vi "Save Settings.vi"(7 "XML File Path":path, 8 "error in (no error)":errorcluster, 10 "Reader Object":refnum<class>, 11 "Scanner Object":refnum<class>) -> (0 "error out":errorcluster)   [LabVIEW 2017, in "File IO.lvclass"]
uses:
  File IO/File IO.lvclass
  Scanners/Scanner/Write Range UI.vi
  File IO/Setup UI.vi
  <vilib>/Utility/xml.llb/Write to XML File(string).vi
  Scanners/Scanner/Scanner.lvclass
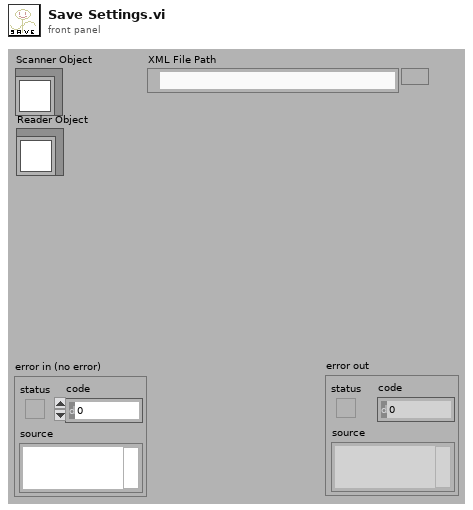
[diagram p1: front panel]
types:
  T1 = cluster{"output cluster":cluster{i32[][], string[]}, "output cluster":cluster{i32[][], string[]}, "output cluster":cluster{i32[][], string[]}, "output cluster":cluster{i32[][], string[]}}
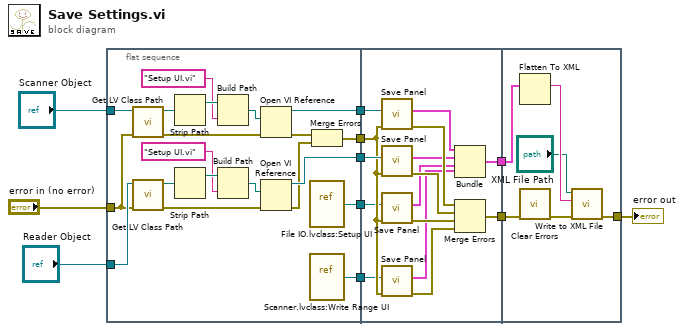
[diagram p0: block diagram]
diagram:
  n1 = flat-sequence {
    tunnel: "Scanner Object" -> [w29]
    tunnel: "Reader Object" -> [w31]
    tunnel: "error in (no error)" -> [w30]
    tunnel: [w28] -> w10
    tunnel: [w27] -> w9
    tunnel: [w26] -> w8
    tunnel: [w23] -> w7
    tunnel: [w22] -> w3
    tunnel: w10 -> [w46]
    tunnel: w9 -> [w45]
    tunnel: w8 -> [w44]
    tunnel: w7 -> [w43]
    tunnel: [w38] -> w6
    tunnel: [w33] -> w5
    tunnel: w3 -> [w32]
    tunnel: w6 -> [w52]
    tunnel: w5 -> [w51]
    tunnel: [w50] -> w4
    frame #0 {
      n2 = call <vilib>:"Get LV Class Path.vi"("error in (no error)"=w30, "object"=w29) -> ("error out"=w17:errorcluster, "class path"=w21:path)  [unwired: 8 out]
      n3 = call <vilib>:"Get LV Class Path.vi"("error in (no error)"=w30, "object"=w31) -> ("error out"=w12:errorcluster, "class path"=w16:path)  [unwired: 8 out]
      n4 = Strip Path(path=w21) -> (stripped path=w20:path)  [unwired: 1 out]
      n5 = Strip Path(path=w16) -> (stripped path=w15:path)  [unwired: 1 out]
      n6 = Build Path(base path=w20, name or relative path="Setup UI.vi") -> (appended path=w18:path)
      n7 = Build Path(base path=w15, name or relative path="Setup UI.vi") -> (appended path=w13:path)
      n8 = Open VI Reference(vi path=w18, error in (no error)=w17) -> (vi reference=w28:refnum<vi>, error out=w25:errorcluster)  [unwired: 4 out]
      n9 = Open VI Reference(vi path=w13, error in (no error)=w12) -> (vi reference=w27:refnum<vi>, error out=w24:errorcluster)  [unwired: 4 out]
      n10 = vi-ref "File IO.lvclass:Setup UI.vi"() -> (w22:refnum<vi>)
      n11 = vi-ref "Scanner.lvclass:Write Range UI.vi"() -> (w23:refnum<vi>)
      n12 = Merge Errors(w25, w24) -> (w26:errorcluster)
    }
    frame #1 {
      n13 = call "Save Panel.vi"("error in (no error)"=w44, "vi reference"=w46) -> ("error out"=w42:errorcluster, "output cluster"=w37:cluster{i32[][], string[]})  [unwired: 8 in]
      n14 = call "Save Panel.vi"("error in (no error)"=w44, "vi reference"=w45) -> ("error out"=w41:errorcluster, "output cluster"=w36:cluster{i32[][], string[]})  [unwired: 8 in]
      n15 = call "Save Panel.vi"("error in (no error)"=w44, "vi reference"=w32) -> ("error out"=w40:errorcluster, "output cluster"=w35:cluster{i32[][], string[]})  [unwired: 8 in]
      n16 = call "Save Panel.vi"("error in (no error)"=w44, "vi reference"=w43) -> ("error out"=w39:errorcluster, "output cluster"=w34:cluster{i32[][], string[]})  [unwired: 8 in]
      n17 = Bundle("output cluster"=w37, "output cluster"=w36, "output cluster"=w35, "output cluster"=w34) -> (w33:T1)  [unwired: 1 in]
      n18 = Merge Errors(w42, w41, w40, w39) -> (w38:errorcluster)
    }
    frame #2 {
      n19 = Flatten To XML(anything=w51) -> (xml string=w49:string)
      n20 = call <vilib>:"Clear Errors.vi"("error in (no error)"=w52) -> ("error out"=w47:errorcluster)  [unwired: 5 in, 1 out]
      n21 = call-poly <vilib>:"Write to XML File.vi"("error in (no error)"=w47, "XML Input"=w49, "XML File Path"="XML File Path") -> ("error out"=w50:errorcluster)  [unwired: 6 in, 2 out]
    }
  }
  "error out" <- w4
